vi "Set State by Position.vi"(8 "error in (no error)":errorcluster, 9 "State":u32, 10 "Position":u32, 11 "Example Application in":refnum<class "Example Application.lvclass">) -> (0 "error out":errorcluster, 3 "Example Application out":refnum<class "Example Application.lvclass">)   [LabVIEW 2015, in "Example Application.lvlib" / "Example Application.lvclass"]
uses:
  Example Application.lvclass
  Example Application.lvclass/Example Application.ctl
  Properties/Example App Properties.lvclass
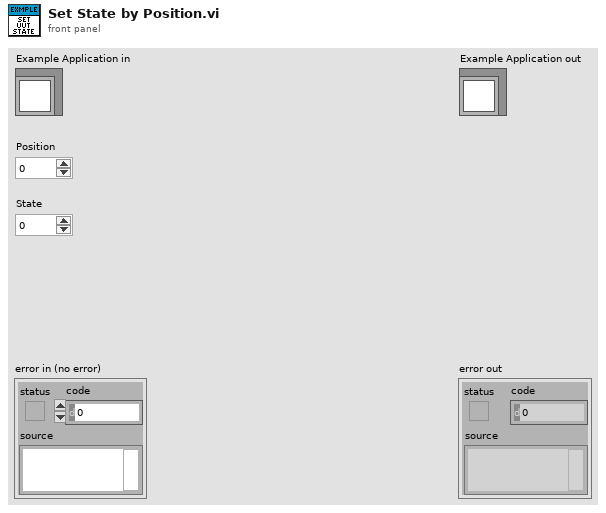
[diagram p1: front panel]
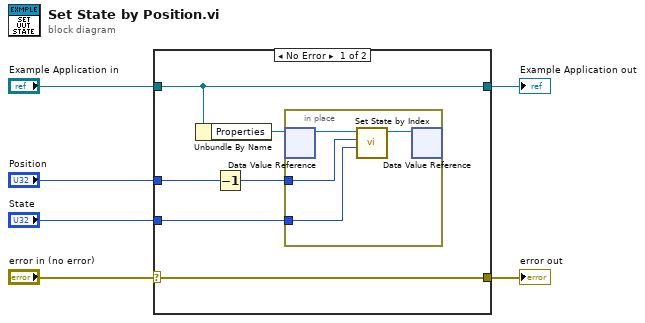
[diagram p0: block diagram]
diagram:
  n1 = case shown="No Error" "error in (no error)" {
    selector: "error in (no error)" -> [w8 w18]
    tunnel: "Example Application in" -> [w7 w17]
    tunnel: "Position" -> [w11 _]
    tunnel: "State" -> [w9 _]
    tunnel: [w8 w18] -> w2
    tunnel: [w7 w17] -> w1
    frame No Error {
      n2 = Unbundle By Name(w7) -> ("Properties"=w12:refnum<data-value>)
      n3 = Decrement(x=w11) -> (x-1=w10:u32)
      n4 = in-place {
        in-place-border: w10 -> [w14]
        in-place-border: w9 -> [w13]
        n5 = in-place-dvr #1(w12) -> (w16:refnum<class "Example App Properties.lvclass">)  [unwired: 1 out]
        n6 = call-dynamic "Set State by Index.vi"("Enum"=w13, "index"=w14, "Example App Properties in"=w16) -> ("Example App Properties out"=w15:refnum<class "Example App Properties.lvclass">)  [unwired: 7 in, 1 out]
        n7 = in-place-dvr #1(w15) -> ()  [unwired: 2 out]
      }
    }
    frame Error {
    }
  }
  "error out" <- w2
  "Example Application out" <- w1
